vi "Write Data to HW.vi"(11 "Custom Device in":refnum<class "Template.lvclass">) -> (0 "error out":errorcluster, 3 "Custom Device out":refnum<class "Template.lvclass">)   [LabVIEW 2026, in "Template.lvlib" / "Template.lvclass"]
uses:
  Template.lvclass
  Template.lvclass/Template.ctl
  <userlib>/Custom Device Interfaces_v1.lvlibp/CustomDeviceAPI/Custom Device API.lvclass
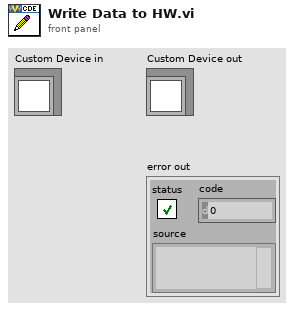
[diagram p1: front panel]
types:
  T1 = cluster{"Data Reference":i32, "Offset":u64, "Length":u64}[]
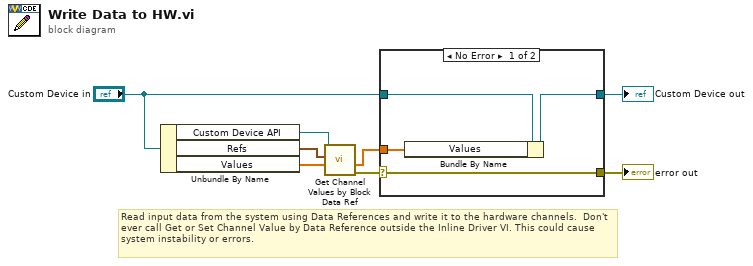
[diagram p0: block diagram]
diagram:
  # "Read input data from the system using Data References and write it to the hardware channels.  Don't ever call Get or Set Channel Value by Data Reference outside the Inline Driver VI. This could cause system instability or errors."
  n1 = Unbundle By Name("Custom Device in") -> ("Custom Device API"=w3:refnum<class "Custom Device API.lvclass">, "Refs"=w2:T1, "Values"=w1:dbl[])
  n2 = call-dynamic "Get Channel Values by Block Data Ref.vi"("Values in"=w1, "Block Data Ref in"=w2, "Custom Device API in"=w3) -> ("error out"=w5:errorcluster, "Values out"=w4:dbl[])  [unwired: 5 in, 2 out]
  n3 = case shown="No Error" w5 {
    selector: w5 -> [w9 w13]
    tunnel: w4 -> [w10 _]
    tunnel: "Custom Device in" -> [w12 w14]
    tunnel: [w11 w14] -> w6
    tunnel: [w9 w13] -> w7
    frame No Error {
      n4 = Bundle By Name(cluster=w12, "Values"=w10) -> (w11:refnum<class "Template.lvclass">)
    }
    frame Error {
    }
  }
  "error out" <- w7
  "Custom Device out" <- w6
